vi "Gen&osc_stepper.vi"() -> ()   [LabVIEW 2018]
uses:
  <vilib>/LabVIEW Interface for Arduino/Type Defs/Board Type.ctl
  <vilib>/LabVIEW Interface for Arduino/Type Defs/Connection Type.ctl
  <instrlib>/LeCroy Wave Series/Public/Data/Read Single Waveform.vi
  <instrlib>/Siglent SDG X Series/Siglent SDG X Series.lvlib
  <instrlib>/LeCroy Wave Series/LeCroy Wave Series.lvlib
  <vilib>/LabVIEW Interface for Arduino/LabVIEW Interface for Arduino.lvlib
panel:
  in  "Tab Control":enum32{"Page 1", "Page 2", "Page 3"}(tab)
  in  "VISA Refnum in":refnum<visa-resource-name>
  in  "Channel (1:Channel 1)":i32(ring)=1 items=["Channel 1"=1, "Channel 2"=2]
  in  "Enable Output (T: Enable)":bool=TRUE
  in  "Amplitude (1.0 Vpp)":dbl=1.0 format="%#.3f"
  in  "Frequency (1000 Hz)":dbl=1000.0 format="%#.6g"
  in  "DC Offset (0.00 V) in":dbl
  in  "Waveform Function (0: Sine) in":u16(ring) items=["Sine", "Square", "Ramp", "DC", "Pulse", "Arb"]
  in  "Phase (0.0 degrees)":dbl=0.002 min=-360.0 max=360.0 format="%#.1g"
  in  "Fall (20 ns)":dbl=2e-08 format="%#.3g"
  in  "Duty (20%)":dbl=20.0 min=0.0001 max=100.0 format="%.4g"
  in  "Delay (0.00 s)":dbl min=-1000000.0 max=1000000.0
  in  "Rise (20 ns)":dbl=2e-08 format="%#.3g"
  in  "True To \ngenerate\n pulse":bool
  out "VISA resource name out":refnum<visa-resource-name>
  out "error out":errorcluster
  in  "format string":string
  out "Output Filename":path
  out "error out 2":errorcluster
  out "Output Directory":path
  in  "File Directory":path
  in  "Filename":string
  out ".not. x?":bool
  in  "stop":bool
  out "Waveform Data":waveform(dbl)(graph)
  in  "Timeout (10000 ms)":u32=10000
  in  "Source (0: Channel 1)":u16(ring) items=["Channel 1", "Channel 2", "Channel 3", "Channel 4", "Memory 1", "Memory 2", "Memory 3", "Memory 4", "Function 1", "Function 2", "Function 3", "Function 4", "Function 5", "Function 6", "Function 7", "Function 8"]
  in  "Perform Auto Setup?":bool
  in  "Reset Scope?":bool
  in  "VISA resource name":refnum<visa-resource-name>
  out "Saved filename":string
  in  "Save Files in Directory":string="D:\\Automation\\Data"
  in  "VISA resource":refnum<visa-resource-name>
  in  "Board Type (Uno)":T1
  in  "error in":errorcluster
  in  "Stepper #":u8
  in  "Stepper Pins":u8[](array[numeric])=[2, 3]
  in  "Control Method":u8(ring)=1 items=["2 Wire (Pulse & Direction)"=1, "2 Wire"=2, "4 Wire"=4, "EasyDriver"=6, "AF Motor Shield (Stepper 1 & 2 Only)"=5]
  in  "Steps for one rotation":i16
  in  "Set Speed (Steps per Second)":i16=100
  in  "Set Acceleration (0 to disable)":i16
  out "Step Angle":dbl
  in  "Step Size":i16
  out "Steps Remaining?":bool
  in  "Baud Rate (115200)":u32=115200
  # "Set PULSE parameters"
  # "In the oscilloscope memory"
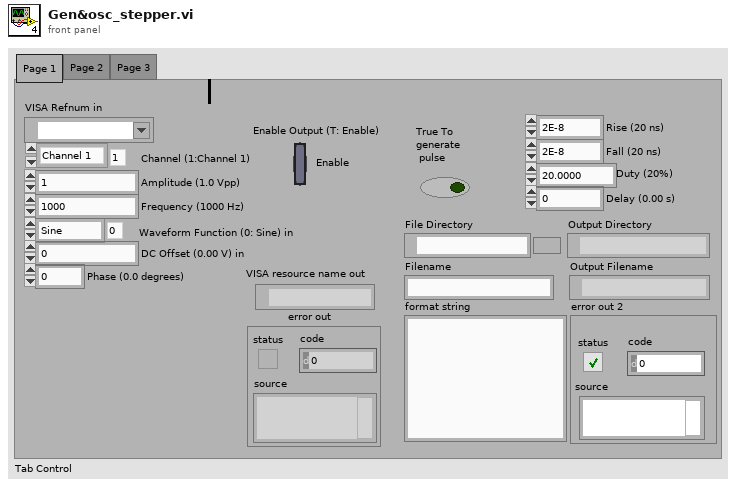
[diagram p1: front panel]
types:
  T1 = typedef "LabVIEW Interface for Arduino.lvlib/Board Type.ctl" = enum16{"Uno", "Dimuelanove w/Atmega 328", "Mega 2560"}
  T2 = typedef "LabVIEW Interface for Arduino.lvlib/Connection Type.ctl" = enum8{"USB / Serial", "XBEE", "BlueSmirf (Bluetooth)"}
  T3 = typedef "LabVIEW Interface for Arduino.lvlib/Arduino Resource.ctl" = cluster{"VISA resource":refnum<visa-resource-name>, "Board Type":T1, "Connection Type":enum8{"USB / Serial"}, "Bytes Per Packet (15)":u8}
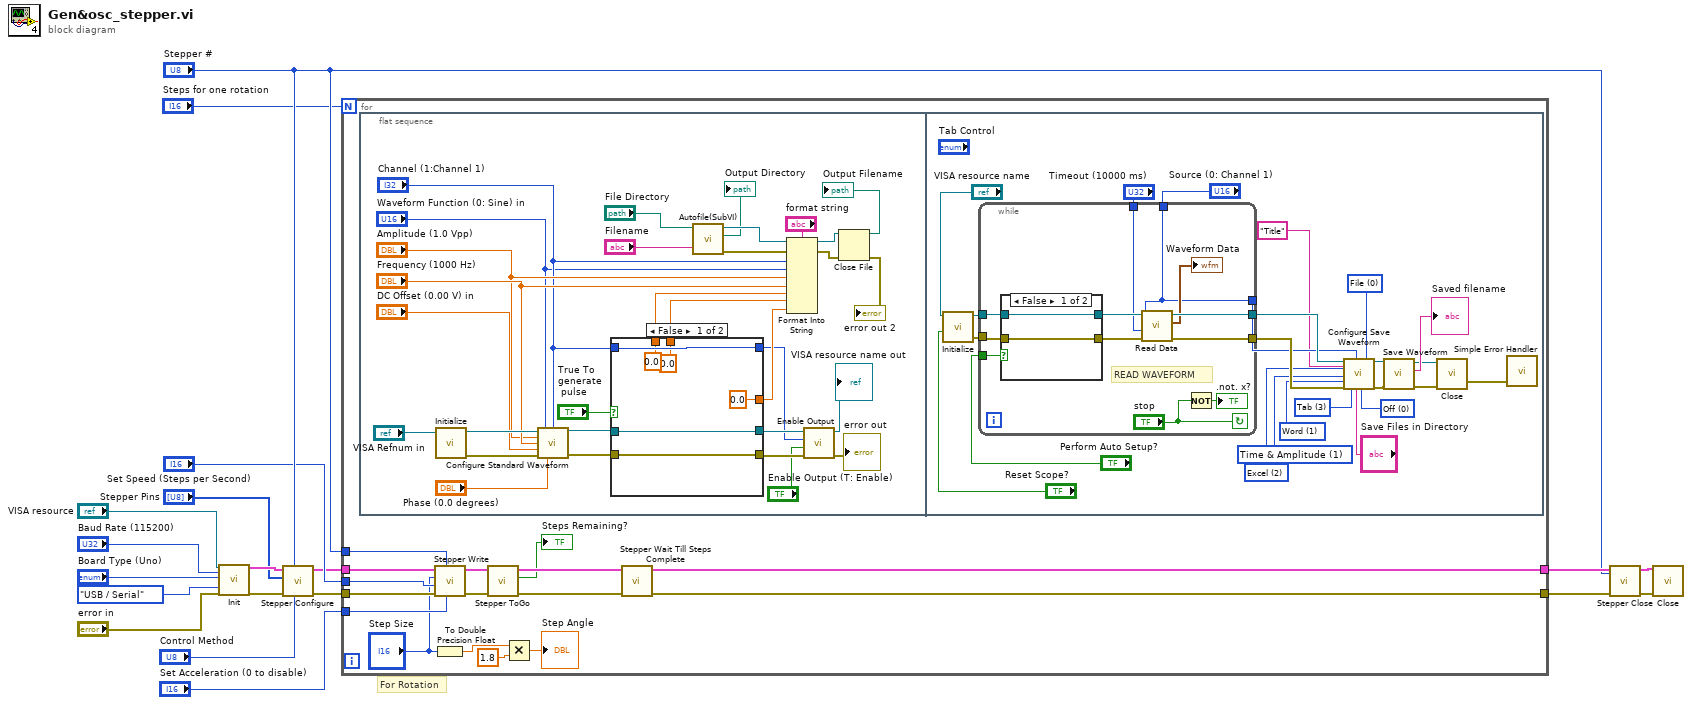
[diagram p0: block diagram]
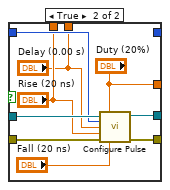
[diagram p2: hidden frame]
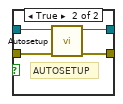
[diagram p3: hidden frame]
diagram:
  # "For Rotation"
  n1 = call <vilib>:"Init.vi"("VISA resource"="VISA resource", "Baud Rate (115200)"="Baud Rate (115200)", "Board Type (Uno)"="Board Type (Uno)", "Connection Type (USB/Serial)"=Connection_Type."USB / Serial", "error in"="error in") -> ("Arduino Resource"=w16:T3, "error out"=w15:errorcluster)  [unwired: 13 in]
  n2 = call <vilib>:"Stepper Configure.vi"("Control Method"="Control Method", "Stepper #"="Stepper #", "error in"=w15, "Stepper Pins"="Stepper Pins", "Arduino Resource"=w16) -> ("error out"=w5:errorcluster, "Arduino Resource Out"=w2:T3)  [unwired: 5 in]
  n3 = for {
    N: "Steps for one rotation" -> [_]
    tunnel: [w32] -> w9
    tunnel: [w31] -> w8
    tunnel: "Set Acceleration (0 to disable)" -> [w30]
    tunnel: "Stepper #" -> [w29]
    tunnel: w5 -> [w28]
    tunnel: "Set Speed (Steps per Second)" -> [w27]
    tunnel: w2 -> [w26]
    n4 = flat-sequence {
      frame #0 {
        n5 = call <instrlib>:"Initialize.vi"("VISA resource name"="VISA Refnum in") -> ("error out"=w60:errorcluster, "VISA resource name out"=w61:refnum<visa-resource-name>)  [unwired: 9 in]
        n6 = call <instrlib>:"Configure Standard Waveform.vi"("VISA resource name"=w61, "Waveform Function (0: Sine)"="Waveform Function (0: Sine) in", "Channel (1:Channel 1)"="Channel (1:Channel 1)", "Amplitude (1.0 Vpp)"="Amplitude (1.0 Vpp)", "Frequency (1000 Hz)"="Frequency (1000 Hz)", "DC Offset (0.00 V)"="DC Offset (0.00 V) in", "error in (no error)"=w60, "Phase (0.0 degrees)"="Phase (0.0 degrees)") -> ("VISA resource name out"=w56:refnum<visa-resource-name>, "error out"=w59:errorcluster)  [unwired: 6 in]
        n7 = case shown="False" "True To \ngenerate\n pulse" {
          tunnel: [w70 w78] -> w65
          tunnel: [w69 w77] -> w64
          tunnel: w56 -> [w70 w76]
          tunnel: w59 -> [w69 w75]
          tunnel: "Channel (1:Channel 1)" -> [_ w74]
          tunnel: "Channel (1:Channel 1)" -> [_ _]
          tunnel: [0.0 ("Duty (20%)") "Duty (20%)"] -> w52
          tunnel: [0.0 ("Rise (20 ns)") "Rise (20 ns)"] -> w44
          tunnel: [0.0 ("Delay (0.00 s)") "Delay (0.00 s)"] -> w43
          frame False {
          }
          frame True {
            n8 = call <instrlib>:"Configure Pulse.vi"("VISA resource name"=w76, "Duty (20%)"="Duty (20%)", "Channel (1:Channel 1)"=w74, "Delay (0.00 s)"="Delay (0.00 s)", "Rise (20 ns)"="Rise (20 ns)", "error in (no error)"=w75, "Fall (20 ns)"="Fall (20 ns)") -> ("VISA resource name out"=w78:refnum<visa-resource-name>, "error out"=w77:errorcluster)  [unwired: 7 in]
          }
        }
        n9 = call "Autofile(SubVI).vi"("Filename"="Filename", "File Directory"="File Directory") -> ("error out"=w39:errorcluster, "Output Directory"=→"Output Directory":path, "Byte Stream File out"=w40:refnum<file>)  [unwired: 7 in]
        n10 = Format Into String(format string="format string", initial string=w40, error in=w39, "Channel (1:Channel 1)", "Waveform Function (0: Sine) in", "Amplitude (1.0 Vpp)", "Frequency (1000 Hz)", w44, w43, w52) -> (resulting string=w51:refnum<file>, error out=w48:errorcluster)
        n11 = call <instrlib>:"Enable Output.vi"("error in (no error)"=w64, "Enable Output (T: Enable)"="Enable Output (T: Enable)", "Channel (1:Channel 1)"="Channel (1:Channel 1)", "VISA resource name"=w65) -> ("error out"=→"error out":errorcluster, "VISA resource name out"=→"VISA resource name out":refnum<visa-resource-name>)  [unwired: 6 in]
        n12 = Close File(refnum=w51, error in=w48) -> (path=→"Output Filename":path, error out=→"error out 2":errorcluster)
      }
      frame #1 {
        w86 = u16 3 items=["Comma", "Space", "Semicolon", "Tab"] ("Delimiter (  0:Comma)")
        w87 = u16 0 items=["Off", "Wrap", "Fill"] ("Auto Save (0:Off")
        w88 = u16 1 items=["Byte", "Word", "Auto"] ("BinarySubFormat (1: Word)")
        w90 = u16 1 items=["Amplitude Only", "Time & Amplitude", "With Header"] ("SubFormat (1: Time & Amplitude)")
        w91 = u16 2 items=["Binary", "ASCII", "Excel", "MATLAB", "MathCad", "WaveML"] ("Format (0: Binary)")
        w92 = u16 0 items=["File", "M1", "M2", "M3", "M4"] ("Destination (0:File)")
        n13 = call <instrlib>:"Initialize.vi"("Reset? (T: Yes)"="Reset Scope?", "VISA resource name"="VISA resource name") -> ("error out"=w100:errorcluster, "VISA resource name out"=w101:refnum<visa-resource-name>)  [unwired: 8 in]
        n14 = while {
          tunnel: [w113] -> w94
          tunnel: [w112] -> w95
          tunnel: "Perform Auto Setup?" -> [w111]
          tunnel: "Source (0: Channel 1)" -> [w104]
          tunnel: w100 -> [w110]
          tunnel: w101 -> [w109]
          tunnel: "Timeout (10000 ms)" -> [w108]
          tunnel: [w104] -> w93
          stop <- "stop" continue-if-true
          # "READ WAVEFORM"
          n15 = case shown="False" w111 {
            tunnel: w110 -> [w116 w121]
            tunnel: w109 -> [w117 w120]
            tunnel: [w117 w119] -> w115
            tunnel: [w116 w118] -> w114
            frame False {
            }
            frame True {
              # "AUTOSETUP"
              n16 = call <instrlib>:"Autosetup.vi"("error in (no error)"=w121, "VISA resource name"=w120) -> ("error out"=w118:errorcluster, "VISA resource name out"=w119:refnum<visa-resource-name>)  [unwired: 8 in]
            }
          }
          n17 = call-poly <instrlib>:"Read Data.vi"("error in (no error)"=w114, "Timeout (10000 ms)"=w108, "Source (0: Channel 1)"=w104, "VISA resource name"=w115) -> ("error out"=w113:errorcluster, "Waveform Data"=→"Waveform Data":waveform(dbl), "VISA resource name out"=w112:refnum<visa-resource-name>)  [unwired: 5 in]
          n18 = Not(x="stop") -> (.not. x?=→".not. x?":bool)
        }
        n19 = call <instrlib>:"Configure Save Waveform.vi"("VISA resource name"=w95, "Trace Title (Title)"="Title", "Format (0: Binary)"=w91, "SubFormat (1: Time & Amplitude)"=w90, "BinarySubFormat (1: Word)"=w88, "error in (no error)"=w94, "Delimiter (  0:Comma)"=w86, "Source (0: Channel 1)"=w93, "Save Files in Directory (D:\\Waveforms)"="Save Files in Directory", "Auto Save (0:Off"=w87, "Destination (0:File)"=w92) -> ("VISA resource name out"=w84:refnum<visa-resource-name>, "error out"=w83:errorcluster)  [unwired: 7 in]
        n20 = call <instrlib>:"Save Waveform.vi"("error in (no error)"=w83, "VISA resource name"=w84) -> ("error out"=w80:errorcluster, "Saved filename"=→"Saved filename":string, "VISA resource name out"=w81:refnum<visa-resource-name>)  [unwired: 7 in]
        n21 = call <vilib>:"Close.vi"("error in (no error)"=w80, "VISA resource name"=w81) -> ("error out"=w103:errorcluster)  [unwired: 9 in]
        n22 = call <vilib>:"Simple Error Handler.vi"("error in (no error)"=w103) -> ()  [unwired: 4 in, 5 out]
      }
    }
    n23 = call <vilib>:"Stepper Write.vi"("Set Acceleration (0 to disable)"=w30, "Stepper #"=w29, "error in"=w28, "Set Speed (Steps per Second)"=w27, "# of Steps to Move"="Step Size", "Arduino Resource"=w26) -> ("error out"=w25:errorcluster, "Arduino Resource Out"=w24:T3)  [unwired: 4 in]
    n24 = To Double Precision Float(number="Step Size") -> (double precision float=w21:dbl)
    n25 = call <vilib>:"Stepper ToGo.vi"("error in"=w25, "Arduino Resource"=w24) -> ("error out"=w35:errorcluster, "Steps Remaining?"=→"Steps Remaining?":bool, "Arduino Resource Out"=w34:T3)  [unwired: 6 in, 1 out]
    n26 = Multiply(x=w21, y=1.8) -> (x*y=→"Step Angle":dbl)
    n27 = call <vilib>:"Stepper Wait Till Steps Complete.vi"("error in"=w35, "Arduino Resource In"=w34) -> ("error out"=w32:errorcluster, "Arduino Resource Out"=w31:T3)  [unwired: 8 in]
  }
  n28 = call <vilib>:"Stepper Close.vi"("Stepper #"="Stepper #", "error in"=w9, "Arduino Resource"=w8) -> ("error out"=w10:errorcluster, "Arduino Resource Out"=w11:T3)  [unwired: 7 in]
  n29 = call <vilib>:"Close.vi"("Arduino Resource"=w11, "error in"=w10) -> ()  [unwired: 13 in, 1 out]
